vi "Propagate Error.vi"(8 "error in (no error)":errorcluster, 11 "Self Actor in":refnum<class "Self Actor.lvclass">) -> (0 "error out":errorcluster, 3 "Self Actor out":refnum<class "Self Actor.lvclass">)   [LabVIEW 2021, in "LVCAM.lvlib" / "Self Actor.lvclass"]
uses:
  Self Actor.lvclass
  Self Actor.lvclass/Self Actor.ctl
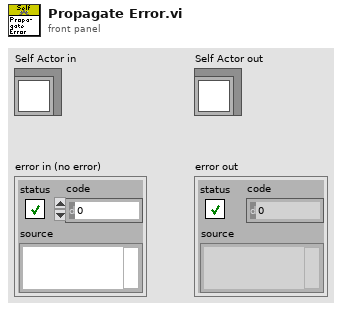
[diagram p1: front panel]
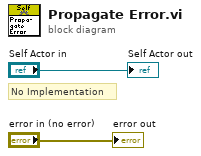
[diagram p0: block diagram]
diagram:
  # "No Implementation"
  "error out" <- "error in (no error)"
  "Self Actor out" <- "Self Actor in"
